vi "Memory.Clear.vi"(8 "error in (no error)":errorcluster, 10 "size":i64 format="%d bytes", 11 "address":u64 format="%016x") -> (0 "error out":errorcluster)   [LabVIEW 2016, in "LabVIEW Memory Manager.lvlib"]
uses:
  LabVIEW Memory Manager.lvlib
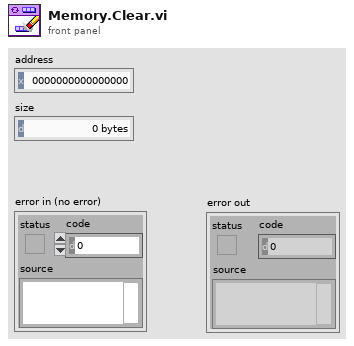
[diagram p1: front panel]
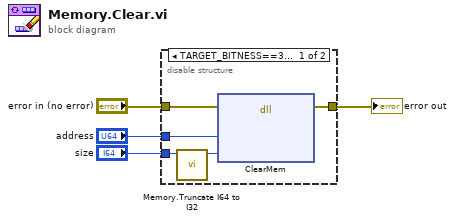
[diagram p0: block diagram]
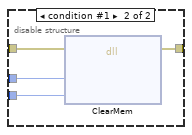
[diagram p2: hidden frame]
diagram:
  n1 = disable-structure shown="TARGET_BITNESS==32, Default" {
    disable-tunnel: "size" -> [w6 w10]
    disable-tunnel: "error in (no error)" -> [w9 w13]
    disable-tunnel: [w8 w12] -> w2
    disable-tunnel: "address" -> [w7 w11]
    frame condition #0 (active) {
      n2 = call "Memory.Truncate I64 to I32.vi"("I64"=w6) -> ("truncated I32"=w5:i32)  [unwired: 10 in]
      n3 = dll-call lib="LabVIEW" fn="ClearMem"(error in=w9, "pointer"=w7, "size"=w5) -> (error out=w8:errorcluster)  [unwired: 5 in, 1 out]
    }
    frame condition #1 {
      n4 = dll-call lib="LabVIEW" fn="ClearMem"(error in=w13, "pointer"=w11, "size"=w10) -> (error out=w12:errorcluster)  [unwired: 5 in, 1 out]
    }
  }
  "error out" <- w2
